vi "1553B_Recv-Beifen.vi"(8 "错误输入（无错误）":errorcluster, 11 "VISA资源名称输入":refnum<visa-resource-name>) -> (0 "error out 2":errorcluster, 3 "VISA资源名称输出":refnum<visa-resource-name>)   [LabVIEW 2012]
uses:
  <vilib>/GPower/VIRegister/Library/Convert/ToU32.vi
  <vilib>/GPower/VIRegister/Library/Convert/ToU8.vi
  <vilib>/GPower/VIRegister/Library/SubVIs/FindRegisterData.vi
  <vilib>/GPower/VIRegister/Library/SubVIs/ReadSub.vi
  <vilib>/GPower/VIRegister/Library/SubVIs/WriteSub.vi
  <vilib>/GPower/VIRegister/Library/QManager/GetRegisterData.vi
  <vilib>/GPower/Error/Library/SetError.vi
  <vilib>/GPower/Error/Library/FilterCodes.vi
  <vilib>/GPower/Error/Library/Filter/FilterMulti.vi
  <vilib>/GPower/VIRegister/Library/QManager/QManagerAction.vi
  <vilib>/GPower/Error/Library/ErrorType.vi
  <vilib>/GPower/Error/Library/SplitAppended.vi
  <vilib>/GPower/Error/Library/SubVIs/ExplanationToError.vi
  <vilib>/GPower/VIRegister/Library/QManager/GetQName.vi
  <vilib>/GPower/VIRegister/Library/QManager/StartQManager.vi
  <vilib>/Utility/error.llb/Trim Whitespace.vi
  <vilib>/dlg_ctls.llb/Space Constant.vi
  <vilib>/Utility/error.llb/Error Code Database.vi
  <vilib>/GPower/Error/Library/SubVIs/SetStatus.vi
  <vilib>/GPower/Error/Library/AppendErrors.vi
  <vilib>/GPower/Error/Library/Append/AppendSingle.vi
  <vilib>/GPower/VIRegister/VIRegister.lvlib
panel:
  out "U8":u8[](array[numeric]) format="%.0x"
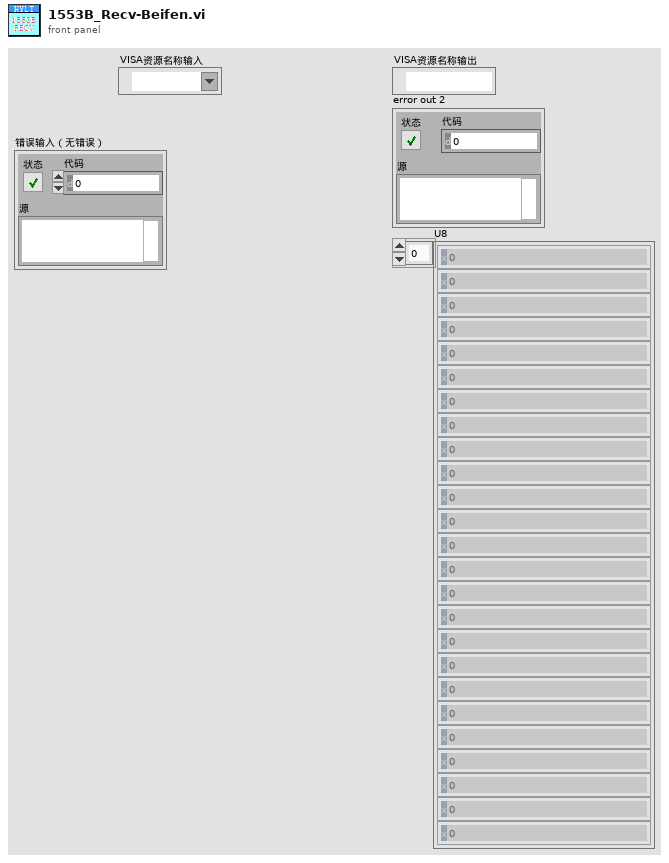
[diagram p1: front panel]
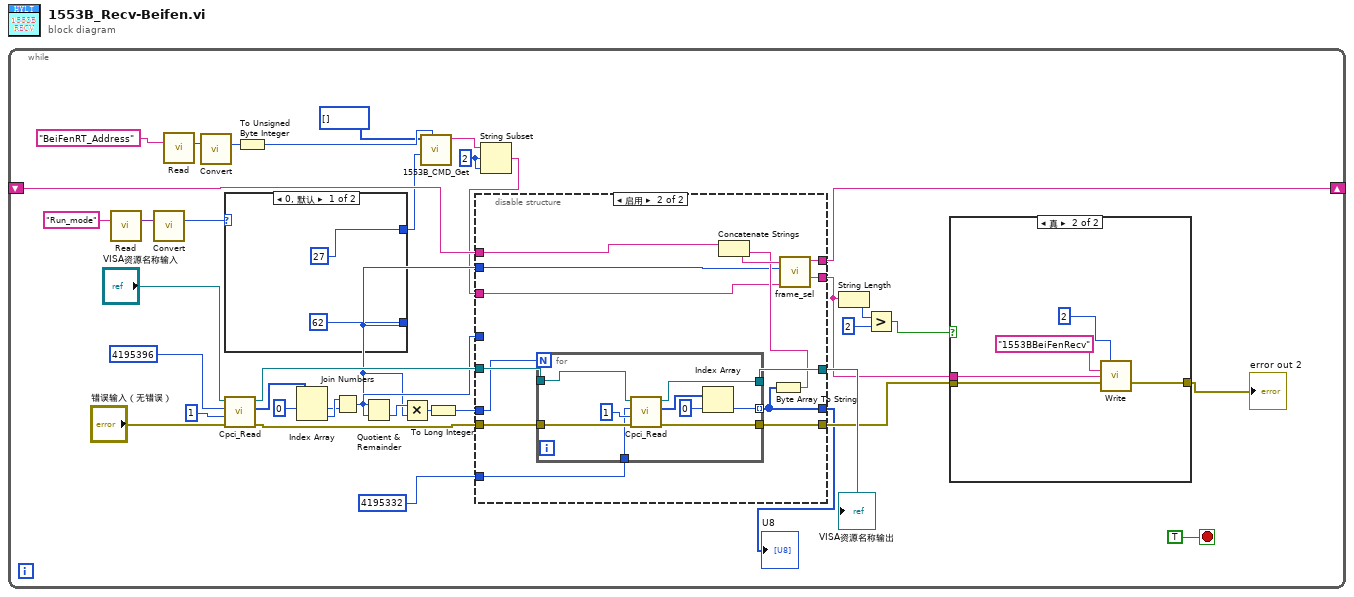
[diagram p0: block diagram]
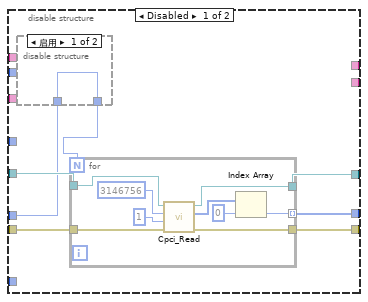
[diagram p3: hidden frame]
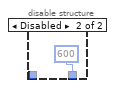
[diagram p4: hidden frame]
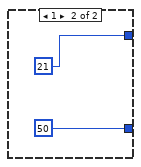
[diagram p5: hidden frame]
diagram:
  n1 = while {
    shift-right: [w19] -> _
    shift-left: _ -> [w18]
    stop <- TRUE stop-if-true
    w12 = 2 ("偏移量(0)")
    n2 = call <vilib>:"Read.vi"("Register name"="Run_mode") -> ("Register value"=w25:variant)  [unwired: 11 in, 3 out]
    n3 = call-poly <vilib>:"Convert.vi"("Register value in"=w25) -> ("Register value out"=w24:u8)  [unwired: 13 in, 1 out]
    n4 = call <vilib>:"Read.vi"("Register name"="BeiFenRT_Address") -> ("Register value"=w8:variant)  [unwired: 11 in, 3 out]
    n5 = call-poly <vilib>:"Convert.vi"("Register value in"=w8) -> ("Register value out"=w9:u32)  [unwired: 13 in, 1 out]
    n6 = case shown="0, 默认" w24 {
      tunnel: [u16 62 ("y") u16 50 ("y")] -> w13
      tunnel: [u16 27 ("y") u16 21 ("y")] -> w4
      frame 0, Default {
      }
      frame 1 {
      }
    }
    n7 = call "Cpci_Read.vi"("错误输入（无错误）"="错误输入（无错误）", "u32_len"=1, "基地址"=u32 4195396 ("y"), "VISA资源名称"="VISA资源名称输入") -> ("错误输出"=w27:errorcluster, "U8"=w35:u8[], "VISA资源名称输出"=w29:refnum<visa-resource-name>)  [unwired: 5 in]
    n8 = To Unsigned Byte Integer(number=w9) -> (unsigned 8bit integer=w10:u8)
    n9 = Index Array(array=w35, index #1=0 ("索引")) -> (element #1=w32:u8, element #2=w33:u8)  [unwired: 1 in]
    n10 = Join Numbers(hi=w33, lo=w32) -> ((hi.lo)=w20:u16)
    n11 = Quotient & Remainder(x=w20, y=w13) -> (floor(x/y)=w31:u16)  [unwired: 1 out]
    n12 = Multiply(x=w31, y=w13) -> (x*y=w30:u16)
    n13 = call "1553B_CMD_Get.vi"("RT地址(默认：01111)"=w10, "字长"=w4, "数据字数组"=u16[] []) -> ("1553B指令"=w11:string)  [unwired: 8 in]
    n14 = To Long Integer(number=w30) -> (32bit integer=w22:i32)
    n15 = String Subset(string=w11, offset (0)=w12, length (rest)=w12) -> (substring=w5:string)
    n16 = disable-structure shown="启用" {
      disable-tunnel: w29 -> [w52 w77]
      disable-tunnel: [w51 w73] -> w1
      disable-tunnel: [w50 w76] -> w28
      disable-tunnel: w27 -> [w49 w75]
      disable-tunnel: [w48 w74] -> w26
      disable-tunnel: w22 -> [w47 w65]
      disable-tunnel: w20 -> [_ _]
      disable-tunnel: [_ w69] -> w17
      disable-tunnel: [_ w68] -> w19
      disable-tunnel: w18 -> [_ w71]
      disable-tunnel: w13 -> [_ w67]
      disable-tunnel: w5 -> [_ w66]
      disable-tunnel: u32 4195332 ("y") -> [_ w64]
      frame Disabled {
        n17 = disable-structure shown="启用" {
          disable-tunnel: w47 -> [w53 _]
          disable-tunnel: [w53 600] -> w46
          frame Enabled {
          }
          frame Disabled {
          }
        }
        n18 = for {
          N: w46 -> [_]
          tunnel: w52 -> [w61]
          tunnel: [w55] -> w51 mode=indexing
          tunnel: [w60] -> w50
          tunnel: w49 -> [w59]
          tunnel: [w58] -> w48
          n19 = call "Cpci_Read.vi"("错误输入（无错误）"=w59, "u32_len"=1, "基地址"=u32 3146756, "VISA资源名称"=w61) -> ("错误输出"=w58:errorcluster, "U8"=w57:u8[], "VISA资源名称输出"=w60:refnum<visa-resource-name>)  [unwired: 5 in]
          n20 = Index Array(array=w57, index=0 ("索引")) -> (element=w55:u8)
        }
      }
      frame Enabled {
        n21 = for {
          N: w65 -> [_]
          tunnel: w77 -> [w85]
          tunnel: [w79] -> w73 mode=indexing
          tunnel: [w84] -> w76
          tunnel: w75 -> [w83]
          tunnel: [w82] -> w74
          tunnel: w64 -> [w78]
          n22 = call "Cpci_Read.vi"("错误输入（无错误）"=w83, "u32_len"=1, "基地址"=w78, "VISA资源名称"=w85) -> ("错误输出"=w82:errorcluster, "U8"=w81:u8[], "VISA资源名称输出"=w84:refnum<visa-resource-name>)  [unwired: 5 in]
          n23 = Index Array(array=w81, index=0 ("索引")) -> (element=w79:u8)
        }
        n24 = Byte Array To String(unsigned byte array=w73) -> (string=w70:string)
        n25 = Concatenate Strings(w71, w70) -> (w72:string)
        n26 = call "frame_sel.vi"("正则表达式"=w66, "帧长"=w67, "输入字符串"=w72) -> ("结果"=w69:string, "剩余"=w68:string)  [unwired: 7 in]
      }
    }
    "VISA资源名称输出" <- w28
    "U8" <- w1
    n27 = String Length(string=w17) -> (length=w16:i32)
    n28 = Greater?(x=w16, y=2) -> (0:w14:bool)
    n29 = case shown="真" w14 {
      tunnel: [w40 w45] -> w38
      tunnel: w26 -> [w40 w44]
      tunnel: w17 -> [_ w43]
      frame False {
      }
      frame True {
        n30 = call <vilib>:"Write.vi"("Timeout"=2, "Register name"="1553BBeiFenRecv", "Register value"=w43, "Error in"=w44) -> ("Error out"=w45:errorcluster)  [unwired: 9 in, 2 out]
      }
    }
    "error out 2" <- w38
  }
